vi "subDataAcquisition_NW348.vi"(4 "# cam.\nframes":u32, 5 "DAQ sampling rate":dbl, 7 "Image file path":path, 8 "error in (no error)":errorcluster caption="Error in (no error)", 9 "DAQ ports":T2, 10 "AO waveform":waveform(dbl), 11 "DO waveform":digitalwaveform[](array[waveform])) -> (0 "error out":errorcluster caption="Error out", 1 "Frame count":i32, 2 "DI waveform":digitalwaveform(waveform)={"t0"=timestamp(0 s since 1904-01-01), "dt"=0.0, "Y"={"transitions"=[], "data"=[]}, "error"={"status"=FALSE, "code"=37421928, "source"=""}}, 3 "AI data":dbl[][](array[numeric]) format="%0.2f")   [LabVIEW 2012]
uses:
  <vilib>/DAQmx/write.llb/DAQmx Write (Analog Wfm 1Chan NSamp).vi
  <vilib>/DAQmx/write.llb/DAQmx Write (Digital 1D Wfm NChan NSamp).vi
  <vilib>/DAQmx/read.llb/DAQmx Read (Analog 2D DBL NChan NSamp).vi
  <vilib>/DAQmx/read.llb/DAQmx Read (Digital Wfm 1Chan NSamp).vi
  <vilib>/DAQmx/write.llb/DAQmx Write (Analog DBL 1Chan 1Samp).vi
  <vilib>/DAQmx/create/channels.llb/DAQmx Create Channel (DO-Digital Output).vi
  <vilib>/DAQmx/create/channels.llb/DAQmx Create Channel (DI-Digital Input).vi
  <vilib>/DAQmx/create/channels.llb/DAQmx Create Channel (AO-Voltage-Basic).vi
  <vilib>/DAQmx/create/channels.llb/DAQmx Create Channel (AI-Voltage-Basic).vi
  <vilib>/Waveform/DWDTOps.llb/DWDT Digital Size.vi
  <vilib>/DAQmx/configure/timing.llb/DAQmx Timing (Sample Clock).vi
  <vilib>/DAQmx/configure/trigger.llb/DAQmx Start Trigger (Digital Edge).vi
  <vilib>/DAQmx/miscellaneous.llb/DAQmx Fill In Error Info.vi
  <vilib>/Waveform/DWDTOps.llb/DWDT Uncompress Digital.vi
panel:
  out "# DO channels":i32
  in  "AI config":T1={"V_max"=10.0, "V_min"=-10.0, "terminal config"=10083} {"terminal config" items=["Default"=-1, "RSE"=10083, "Differential"=10106, "Pseudodifferential"=12529]}
  in  "AO config":T1={"V_max"=2.0, "V_min"=-2.0, "terminal config"=10083} {"terminal config" items=["Default"=-1, "RSE"=10083, "Differential"=10106, "Pseudodifferential"=12529]}
  in  "time after \npre-pulse (ms)":u32=10
  # "First channel of DO\nis camera trigger"
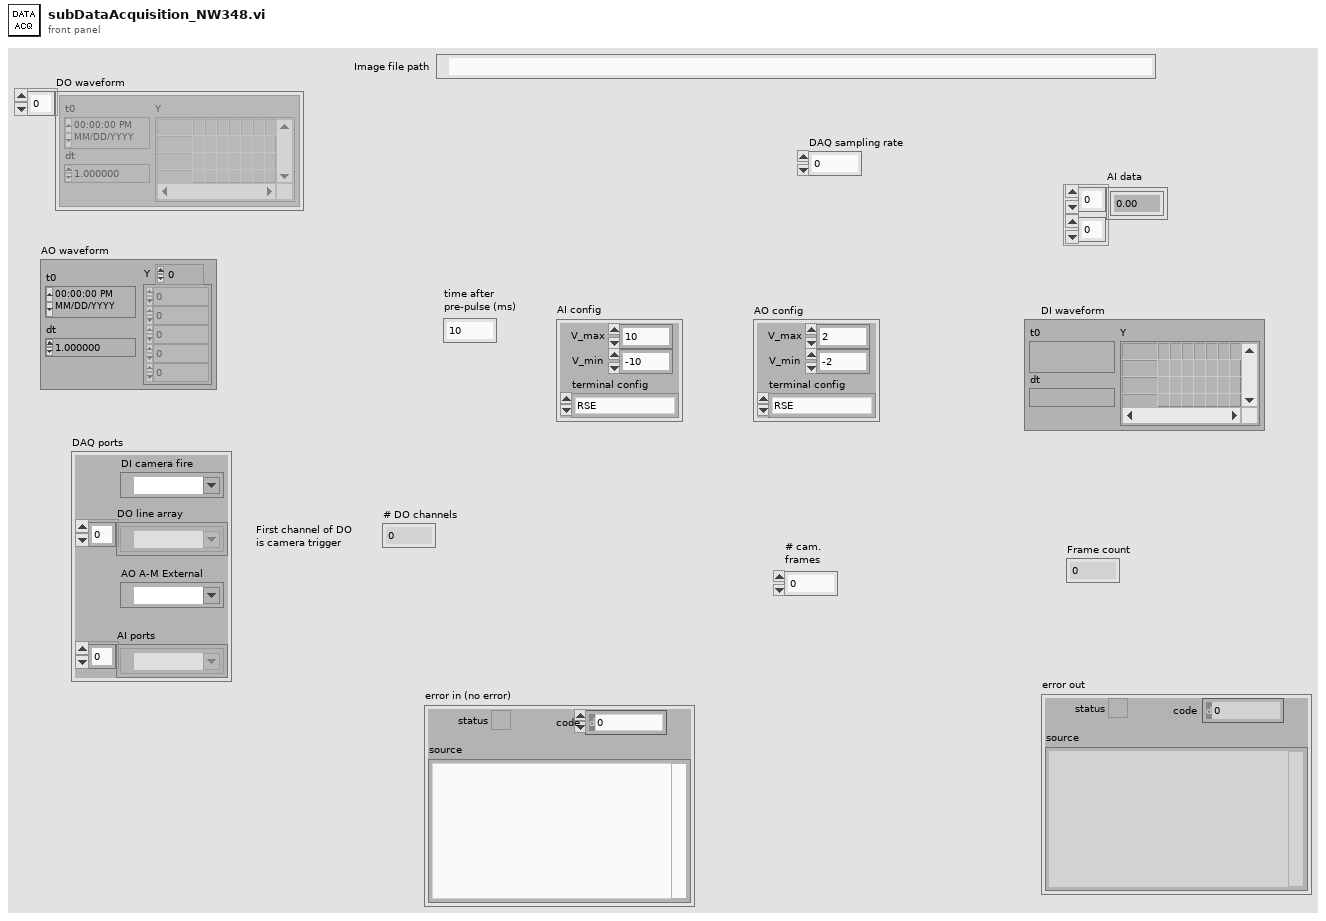
[diagram p1: front panel]
types:
  T1 = cluster{"V_max":dbl, "V_min":dbl, "terminal config":i32}
  T2 = cluster{"DI camera fire":tag, "DO line array":tag[], "AO A-M External":tag, "AI ports":tag[]}
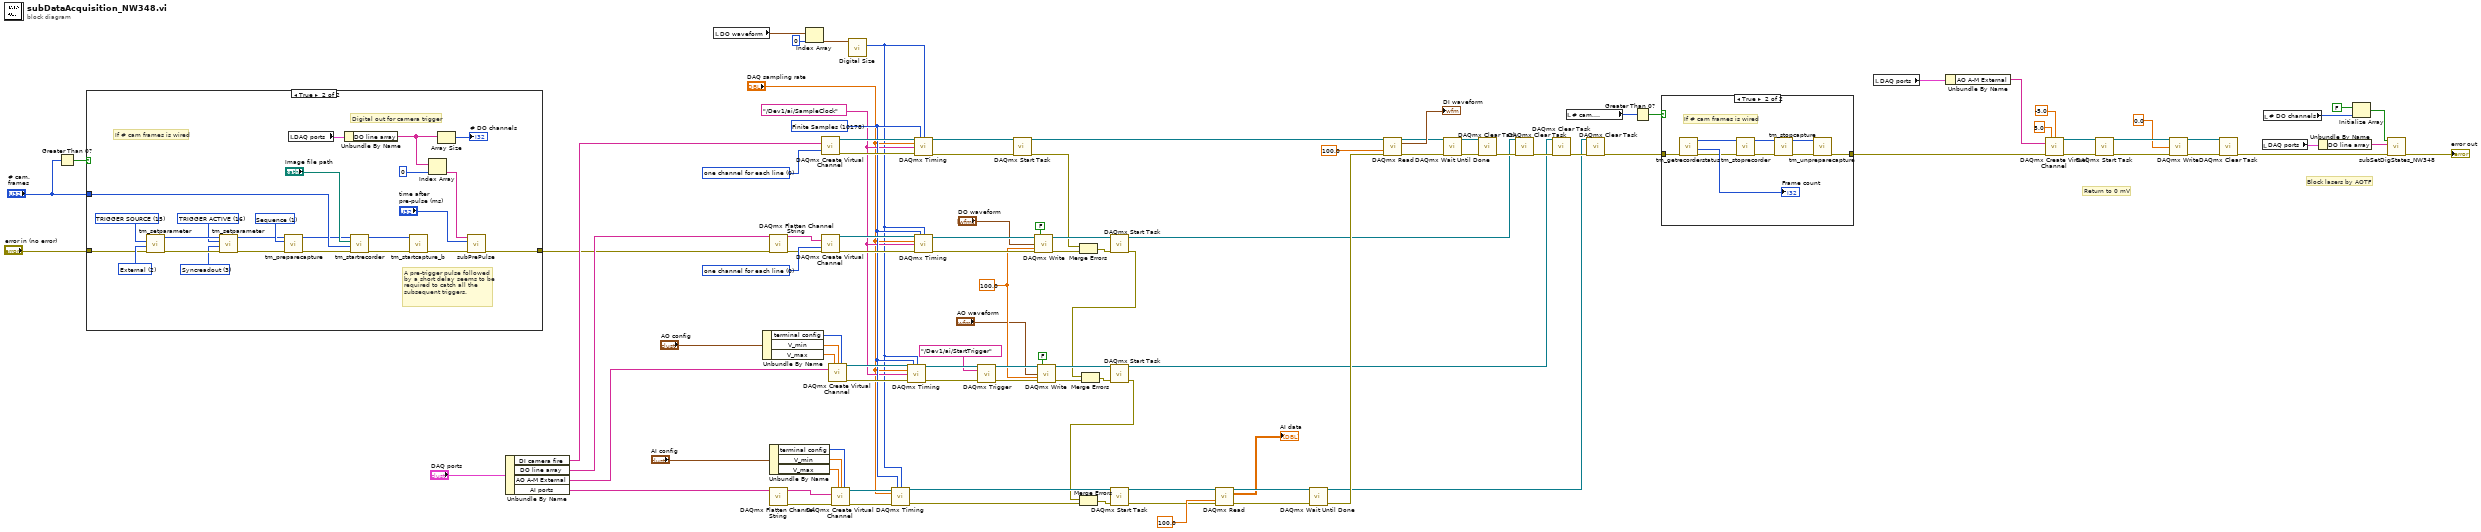
[diagram p0: block diagram]
diagram:
  w66 = 0 items=["one channel for each line", "one channel for all lines"] ("line grouping")
  w63 = 10178 items=["Finite Samples"=10178, "Continuous Samples"=10123, "Hardware Timed Single Point"=12522] ("sample mode")
  w62 = tag "/Dev1/ai/SampleClock" ("source")
  w61 = 100.0 ("timeout")
  w95 = 0 items=["one channel for each line", "one channel for all lines"] ("line grouping")
  # "Block lasers by AOTF"
  # "Return to 0 mV"
  n1 = Greater Than 0?(x="# cam.\nframes") -> (x > 0?=w5:bool)
  n2 = case shown="True" w5 {
    tunnel: "# cam.\nframes" -> [_ w131]
    tunnel: "error in (no error)" -> [w107 w115]
    tunnel: [w107 w113] -> w1
    frame False {
      # "If # cam frames is not wired, then DO NOT run camera; ONLY run DAQ"
    }
    frame True {
      w118 = 3 items=["Edge"=1, "Level"=2, "Syncreadout"=3] ("Trigger Source")
      w119 = 16 items=["BINNING"=1, "BITS PER CHANNEL"=2, "ACTIVE VIEW INDEX"=3, "CCD MODE"=4, "SENSOR MODE"=5, "READOUT MODE"=6, "EXPOSURE TIME"=7, "CONTRAST GAIN"=8, "CONTRAST OFFSET"=9, "LIGHT MODE"=10, "SENSITIVITY"=11, "WHITE BALANCE"=12, "PHOTON IMAGING MODE"=13, "HIGH DYNAMIC RANGE MODE"=14, "TRIGGER SOURCE"=15, "TRIGGER ACTIVE"=16, "TRIGGER MODE"=17, "TRIGGER POLARITY"=18, "TRIGGER GLOBAL EXPOSURE"=19, "FIRST TRIGGER BEHAVIOR"=20, "TRIGGER TIMES"=21, "OUTPUT TRIGGER POLARITY"=22, "OUTPUT TRIGGER DELAY"=23, "OUTPUT TRIGGER PERIOD"=24, "TEMPERATURE"=25, "TEMPERATURE TARGET"=26, "SENSOR COOLER FAN"=27, "MECHANICAL SHUTTER"=28, "BACK FOCUS POSITION"=29, "FRAMEBUNDLE MODE"=30, "FRAMEBUNDLE NUMBER"=31, "LINEBUNDLE HEIGHT"=32, "TRIGGER CONNECTOR"=33, "IMAGE PIXEL TYPE"=34] ("Parameter")
      w122 = 2 items=["Internal"=1, "External"=2, "Software"=3] ("Trigger Source")
      w123 = 15 items=["BINNING"=1, "BITS PER CHANNEL"=2, "ACTIVE VIEW INDEX"=3, "CCD MODE"=4, "SENSOR MODE"=5, "READOUT MODE"=6, "EXPOSURE TIME"=7, "CONTRAST GAIN"=8, "CONTRAST OFFSET"=9, "LIGHT MODE"=10, "SENSITIVITY"=11, "WHITE BALANCE"=12, "PHOTON IMAGING MODE"=13, "HIGH DYNAMIC RANGE MODE"=14, "TRIGGER SOURCE"=15, "TRIGGER ACTIVE"=16, "TRIGGER MODE"=17, "TRIGGER POLARITY"=18, "TRIGGER GLOBAL EXPOSURE"=19, "FIRST TRIGGER BEHAVIOR"=20, "TRIGGER TIMES"=21, "OUTPUT TRIGGER POLARITY"=22, "OUTPUT TRIGGER DELAY"=23, "OUTPUT TRIGGER PERIOD"=24, "TEMPERATURE"=25, "TEMPERATURE TARGET"=26, "SENSOR COOLER FAN"=27, "MECHANICAL SHUTTER"=28, "BACK FOCUS POSITION"=29, "FRAMEBUNDLE MODE"=30, "FRAMEBUNDLE NUMBER"=31, "LINEBUNDLE HEIGHT"=32, "TRIGGER CONNECTOR"=33, "IMAGE PIXEL TYPE"=34] ("Parameter")
      w124 = 1 items=["Snap", "Sequence"] ("Capture mode")
      # "If # cam frames is wired"
      # "Digital out for camera trigger"
      # "A pre-trigger pulse followed\nby a short delay seems to be required to catch all the subsequent triggers."
      n3 = call <userlib>:"tm_setparameter.vi"("error in (no error)"=w115, "Value in"=w122, "Parameter"=w123) -> ("error out"=w120:errorcluster, "Handle out"=w121:u32)  [unwired: 7 in]
      n4 = call <userlib>:"tm_setparameter.vi"("error in (no error)"=w120, "Value in"=w118, "Parameter"=w119, "Handle in"=w121) -> ("error out"=w117:errorcluster, "Handle out"=w116:u32)  [unwired: 6 in]
      n5 = call <userlib>:"tm_preparecapture.vi"("error in (no error)"=w117, "Capture mode"=w124, "Handle in"=w116) -> ("error out"=w128:errorcluster, "Handle out"=w126:u32)  [unwired: 5 in, 2 out]
      n6 = local read "DAQ ports"() -> (w110:T2)
      n7 = Unbundle By Name(w110) -> ("DO line array"=w109:tag[])
      n8 = call <userlib>:"tm_startrecorder.vi"("error in (no error)"=w128, "frames"=w131, "File"="Image file path", "Handle in"=w126) -> ("error out"=w127:errorcluster, "Handle out"=w125:u32)  [unwired: 6 in]
      n9 = call <userlib>:"tm_startcapture_b.vi"("error in (no error)"=w127, "Handle in"=w125) -> ("error out"=w114:errorcluster)  [unwired: 8 in, 1 out]
      n10 = Index Array(array=w109, index=0) -> (element=w111:tag)
      n11 = Array Size(array=w109) -> (size(s)=→"# DO channels":i32)
      n12 = call "subPrePulse.vi"("Error in (no error)"=w114, "time after pulse (ms)"="time after \npre-pulse (ms)", "DO camera"=w111) -> ("Error out"=w113:errorcluster)  [unwired: 8 in]
    }
  }
  n13 = Unbundle By Name("DAQ ports") -> ("DI camera fire"=w58:tag, "DO line array"=w14:tag[], "AO A-M External"=w13:tag, "AI ports"=w15:tag[])
  n14 = local read "DO waveform"() -> (w19:digitalwaveform[])
  n15 = Unbundle By Name("AO config") -> ("terminal config"=w75:i32, "V_min"=w74:dbl, "V_max"=w73:dbl)
  n16 = call <vilib>:"DAQmx Flatten Channel String.vi"("names in"=w14, "error in"=w1) -> ("names out"=w93:string, "error out"=w92:errorcluster)  [unwired: 12 in]
  n17 = Unbundle By Name("AI config") -> ("terminal config"=w72:i32, "V_min"=w71:dbl, "V_max"=w70:dbl)
  n18 = call <vilib>:"DAQmx Flatten Channel String.vi"("names in"=w15) -> ("names out"=w84:string, "error out"=w86:errorcluster)  [unwired: 13 in]
  n19 = Index Array(array=w19, index=0) -> (element=w17:digitalwaveform)
  n20 = call-poly <vilib>:"DAQmx Create Virtual Channel.vi"("lines"=w58, "line grouping"=w66) -> ("task out"=w65:refnum<k21>, "error out"=w64:errorcluster)  [unwired: 12 in]
  n21 = call-poly <vilib>:"DAQmx Create Virtual Channel.vi"("lines"=w93, "line grouping"=w95, "error in"=w92) -> ("task out"=w94:refnum<k21>, "error out"=w85:errorcluster)  [unwired: 11 in]
  n22 = call-poly <vilib>:"DAQmx Create Virtual Channel.vi"("maximum value"=w73, "minimum value"=w74, "output terminal configuration"=w75, "physical channels"=w13) -> ("task out"=w83:refnum<k21>, "error out"=w77:errorcluster)  [unwired: 10 in]
  n23 = call-poly <vilib>:"DAQmx Create Virtual Channel.vi"("maximum value"=w70, "minimum value"=w71, "input terminal configuration"=w72, "physical channels"=w84, "error in"=w86) -> ("task out"=w88:refnum<k21>, "error out"=w87:errorcluster)  [unwired: 9 in]
  n24 = call-poly <vilib>:"Digital Size.vi"("digital waveform in"=w17) -> ("number of samples"=w16:i32)  [unwired: 7 in, 3 out]
  n25 = call-poly <vilib>:"DAQmx Timing.vi"("task/channels in"=w88, "sample mode"=w63, "samples per channel"=w16, "rate"="DAQ sampling rate", "error in"=w87) -> ("task out"=w91:refnum<k21>, "error out"=w51:errorcluster)  [unwired: 9 in]
  n26 = call-poly <vilib>:"DAQmx Timing.vi"("task/channels in"=w83, "sample mode"=w63, "samples per channel"=w16, "rate"="DAQ sampling rate", "source"=w62, "error in"=w77) -> ("task out"=w78:refnum<k21>, "error out"=w79:errorcluster)  [unwired: 8 in]
  n27 = call-poly <vilib>:"DAQmx Timing.vi"("task/channels in"=w65, "sample mode"=w63, "samples per channel"=w16, "rate"="DAQ sampling rate", "source"=w62, "error in"=w64) -> ("task out"=w59:refnum<k21>, "error out"=w60:errorcluster)  [unwired: 8 in]
  n28 = call-poly <vilib>:"DAQmx Timing.vi"("task/channels in"=w94, "sample mode"=w63, "samples per channel"=w16, "rate"="DAQ sampling rate", "source"=w62, "error in"=w85) -> ("task out"=w68:refnum<k21>, "error out"=w67:errorcluster)  [unwired: 8 in]
  n29 = call-poly <vilib>:"DAQmx Trigger.vi"("task/channels in"=w78, "source"=tag "/Dev1/ai/StartTrigger", "error in"=w79) -> ("task out"=w81:refnum<k21>, "error out"=w80:errorcluster)  [unwired: 11 in]
  n30 = call <vilib>:"DAQmx Start Task.vi"("task/channels in"=w59, "error in"=w60) -> ("task out"=w43:refnum<k21>, "error out"=w52:errorcluster)  [unwired: 12 in]
  n31 = call-poly <vilib>:"DAQmx Write.vi"("task/channels in"=w68, "auto start"=FALSE, "data"="DO waveform", "timeout"=w61, "error in"=w67) -> ("task out"=w90:refnum<k21>, "error out"=w56:errorcluster)  [unwired: 8 in, 1 out]
  n32 = call-poly <vilib>:"DAQmx Write.vi"("task/channels in"=w81, "auto start"=FALSE, "data"="AO waveform", "timeout"=w61, "error in"=w80) -> ("task out"=w82:refnum<k21>, "error out"=w55:errorcluster)  [unwired: 8 in, 1 out]
  n33 = Merge Errors(w52, w56) -> (w57:errorcluster)
  n34 = call <vilib>:"DAQmx Start Task.vi"("task/channels in"=w90, "error in"=w57) -> ("task out"=w28:refnum<k21>, "error out"=w53:errorcluster)  [unwired: 12 in]
  n35 = Merge Errors(w53, w55) -> (w54:errorcluster)
  n36 = call <vilib>:"DAQmx Start Task.vi"("task/channels in"=w82, "error in"=w54) -> ("task out"=w27:refnum<k21>, "error out"=w49:errorcluster)  [unwired: 12 in]
  n37 = Merge Errors(w49, w51) -> (w50:errorcluster)
  n38 = call <vilib>:"DAQmx Start Task.vi"("task/channels in"=w91, "error in"=w50) -> ("task out"=w44:refnum<k21>, "error out"=w35:errorcluster)  [unwired: 12 in]
  n39 = call-poly <vilib>:"DAQmx Read.vi"("task/channels in"=w44, "timeout"=100.0, "error in"=w35) -> ("task out"=w45:refnum<k21>, "data"=→"AI data":dbl[][], "error out"=w34:errorcluster)  [unwired: 10 in]
  n40 = call <vilib>:"DAQmx Wait Until Done.vi"("task/channels in"=w45, "error in"=w34) -> ("task out"=w26:refnum<k21>, "error out"=w33:errorcluster)  [unwired: 12 in]
  n41 = call-poly <vilib>:"DAQmx Read.vi"("task/channels in"=w43, "timeout"=100.0, "error in"=w33) -> ("task out"=w31:refnum<k21>, "data"=→"DI waveform":digitalwaveform, "error out"=w32:errorcluster)  [unwired: 10 in]
  n42 = call <vilib>:"DAQmx Wait Until Done.vi"("task/channels in"=w31, "error in"=w32) -> ("task out"=w30:refnum<k21>, "error out"=w29:errorcluster)  [unwired: 12 in]
  n43 = call <vilib>:"DAQmx Clear Task.vi"("task in"=w30, "error in"=w29) -> ("error out"=w47:errorcluster)  [unwired: 13 in]
  n44 = call <vilib>:"DAQmx Clear Task.vi"("task in"=w28, "error in"=w47) -> ("error out"=w46:errorcluster)  [unwired: 13 in]
  n45 = call <vilib>:"DAQmx Clear Task.vi"("task in"=w27, "error in"=w46) -> ("error out"=w48:errorcluster)  [unwired: 13 in]
  n46 = local read "# cam.\nframes"() -> (w2:u32)
  n47 = call <vilib>:"DAQmx Clear Task.vi"("task in"=w26, "error in"=w48) -> ("error out"=w25:errorcluster)  [unwired: 13 in]
  n48 = Greater Than 0?(x=w2) -> (x > 0?=w3:bool)
  n49 = case shown="True" w3 {
    tunnel: w25 -> [w132 w134]
    tunnel: [w132 w133] -> w24
    frame False {
      # "If # cam frames is not wired, \nthen DO NOT run camera"
    }
    frame True {
      # "If # cam frames is wired"
      n50 = call <userlib>:"tm_getrecorderstatus.vi"("error in (no error)"=w134) -> ("error out"=w138:errorcluster, "Count"=→"Frame count":i32, "Handle"=w137:u32)  [unwired: 7 in, 1 out]
      n51 = call <userlib>:"tm_stoprecorder.vi"("error in (no error)"=w138, "Handle in"=w137) -> ("error out"=w136:errorcluster)  [unwired: 8 in, 1 out]
      n52 = call <userlib>:"tm_stopcapture.vi"("error in (no error)"=w136, "Handle in"=w137) -> ("error out"=w135:errorcluster)  [unwired: 8 in, 1 out]
      n53 = call <userlib>:"tm_unpreparecapture.vi"("error in (no error)"=w135, "Handle in"=w137) -> ("error out"=w133:errorcluster)  [unwired: 8 in, 1 out]
    }
  }
  n54 = local read "DAQ ports"() -> (w36:T2)
  n55 = Unbundle By Name(w36) -> ("AO A-M External"=w98:tag)
  n56 = call-poly <vilib>:"DAQmx Create Virtual Channel.vi"("maximum value"=5.0, "minimum value"=-5.0, "physical channels"=w98, "error in"=w24) -> ("task out"=w104:refnum<k21>, "error out"=w103:errorcluster)  [unwired: 5 in, 5 out]
  n57 = call <vilib>:"DAQmx Start Task.vi"("task/channels in"=w104, "error in"=w103) -> ("task out"=w105:refnum<k21>, "error out"=w106:errorcluster)  [unwired: 12 out]
  n58 = call-poly <vilib>:"DAQmx Write.vi"("task/channels in"=w105, "data"=0.0 ("maximum value"), "error in"=w106) -> ("task out"=w99:refnum<k21>, "error out"=w100:errorcluster)  [unwired: 1 in, 10 out]
  n59 = call <vilib>:"DAQmx Clear Task.vi"("task in"=w99, "error in"=w100) -> ("error out"=w7:errorcluster)  [unwired: 13 out]
  n60 = local read "DAQ ports"() -> (w12:T2)
  n61 = local read "# DO channels"() -> (w10:i32)
  n62 = Unbundle By Name(w12) -> ("DO line array"=w11:tag[])
  n63 = Initialize Array(FALSE, w10) -> (w8:bool[])
  n64 = call "subSetDigStates_NW348.vi"("Error in (no error)"=w7, "Digital line array"=w11, "Digital state array"=w8) -> ("Error out"=→"error out":errorcluster)  [unwired: 8 in]
